vi "Wait Scan2_Rf.vi"(8 "error in (no error)":errorcluster, 11 "Data In":T2) -> (0 "error out":errorcluster, 1 "States":T1, 3 "Data Out":T2)   [LabVIEW 2014]
doc: "Use this template to build a standard state machine design pattern. Each state executes code and determines which state to transition to. Contrast this design pattern with the User Interface Event Handler pattern, in which code executes in response to user actions. Contrast this design pattern also with the Queued Message Handler pattern, in which each message handling code can queue zero or more new messages.\nNote: This template does not contain the most recent programming guidelines recommended by National Instruments. For a complete, project-based implementation of the Standard State Machine pattern, use the Create Project dialog box instead of this template."
uses:
  controls/Data.ctl
  controls/State.ctl
  controls/Wait Scan2 States.ctl
panel:
  # "日期"
  # "機種名稱"
  # "機種代號"
  # "商品條碼"
  # "台"
  # "OK"
  # "NG"
  # "台"
  # "總計"
  # "台"
  # "日期"
  # "機種名稱"
  # "機種代號"
  # "商品條碼"
  # "台"
  # "OK"
  # "NG"
  # "台"
  # "總計"
  # "台"
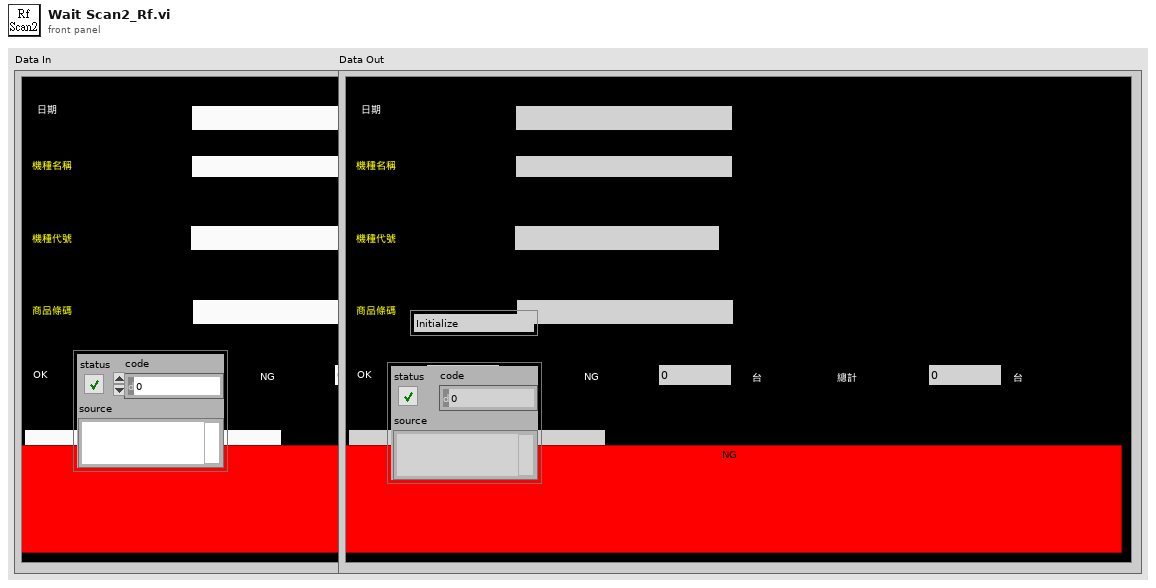
[diagram p1: front panel]
types:
  T1 = typedef "State.ctl" = enum16{"Initialize", "Wait for Scan", "State 1", "State 2", "NG", "NG1", "OK", "OKNG", "Exit"}
  T2 = typedef "Data.ctl" = cluster{"Date":string, "BarCode1":string, "BarCode2":string, "BarCode3":string, "Message":string, "OK Count":u16, "NG Count":u16, "Total Count":u16, "ModelData":string[][], "OK&NG":bool, "COM1":refnum<visa-resource-name>, "COM2":refnum<visa-resource-name>, "IO":i32, "Time":u32, "TCP":refnum<k5>, "TCP 2":refnum<k5>}
  T3 = typedef "Wait Scan2 States.ctl" = enum16{"Initialize", "Step1", "Step2", "Step3", "Step4", "Step5", "Stop"}
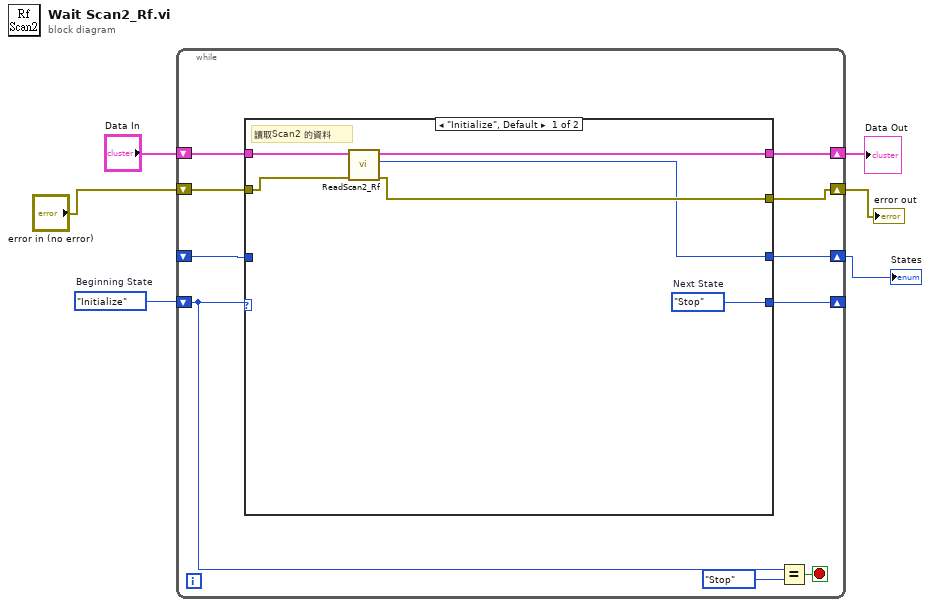
[diagram p0: block diagram]
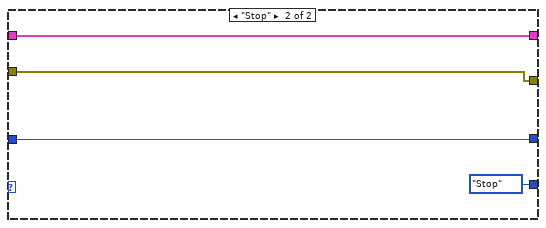
[diagram p2: hidden frame]
diagram:
  w6 = Wait_Scan2_States."Initialize"  # Beginning State
  n1 = while {
    shift-right: [w13] -> _
    shift-left: w6 -> [w14]
    shift-right: [w11] -> w2
    shift-left: "Data In" -> [w12]
    shift-right: [w9] -> w3
    shift-left: "error in (no error)" -> [w10]
    shift-right: [w8] -> w1
    shift-left: _ -> [w7]
    stop <- w16 stop-if-true
    n2 = case shown="\"Initialize\", Default" w14 {
      tunnel: [w22 Wait_Scan2_States."Stop" ("Next State")] -> w13
      tunnel: w12 -> [w21 w25]
      tunnel: [w20 w25] -> w11
      tunnel: w10 -> [w19 w24]
      tunnel: [w18 w24] -> w9
      tunnel: [w17 w23] -> w8
      tunnel: w7 -> [_ w23]
      frame "Initialize", Default {
        w22 = Wait_Scan2_States."Stop"  # Next State
        # "讀取Scan2 的資料"
        n3 = call "ReadScan2_Rf.vi"("error in (no error)"=w19, "Data In"=w21) -> ("error out"=w18:errorcluster, "States"=w17:T1, "Data Out"=w20:T2)  [unwired: 6 in, 1 out]
      }
      frame "Stop" {
      }
    }
    n4 = Equal?(x=w14, y=Wait_Scan2_States."Stop" ("States")) -> (x = y?=w16:bool)
  }
  "Data Out" <- w2
  "error out" <- w3
  "States" <- w1
